vi "GUI_2.vi"() -> ()   [LabVIEW 2023]
uses:
  <vilib>/addons/database/Connection.llb/DB Tools Open Connec (String).vi
  <vilib>/addons/database/Connection.llb/Conn Execute.vi
  <vilib>/addons/database/Recordset.llb/Rec Destroy - Connection.vi
  <vilib>/Instr/_visa.llb/VISA Configure Serial Port (Instr).vi
  <vilib>/addons/database/NI_Database_API.lvlib
panel:
  out "10 V LED":bool
  out "5 V LED":bool
  out "2.5 V LED":bool
  out "1 V LED":bool
  out "10 mV LED":bool
  out "Waveform Graph 2":dbl[](graph)
  in  "stop 2":bool
  out "concatenated string":string
  in  "Unidades":string(combo)
  in  "Canal":enum32{"Item 0", "Item 1"}(radio)
  in  "Guardar":bool
  in  "Autor":string
  out "index":dbl
  out "InicialArr":dbl[](array[numeric])
  out "value":dbl
  out "Canal1":bool
  out "Canal2":bool
  in  "VISA resource name":refnum<visa-resource-name>
  in  "stop":bool
  in  "10 V":bool
  in  "5 V":bool
  in  "2.5 V":bool
  in  "1 V":bool
  in  "10 mV":bool
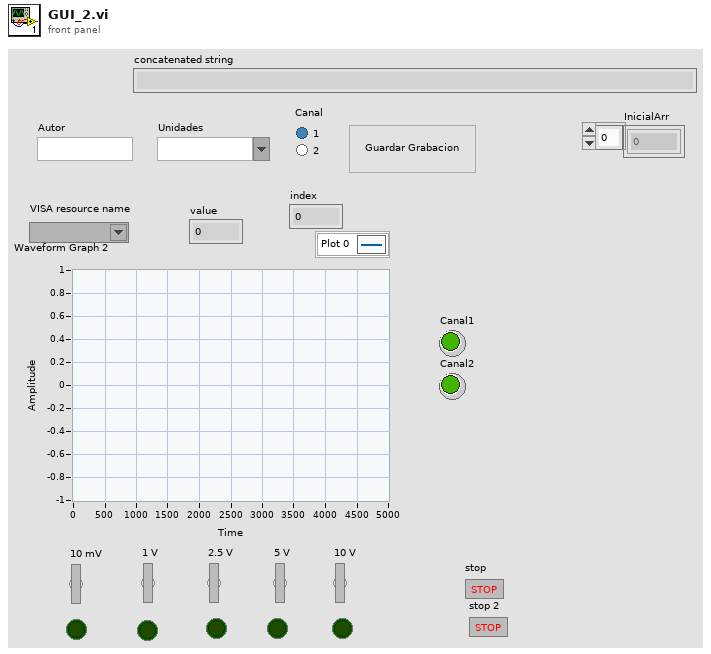
[diagram p1: front panel]
types:
  T1 = typedef "NI_Database_API.lvlib/Conn ObjectReference.ctl" = refnum<k1>
  T2 = typedef "NI_Database_API.lvlib/Rec ObjectReference.ctl" = refnum<k1>
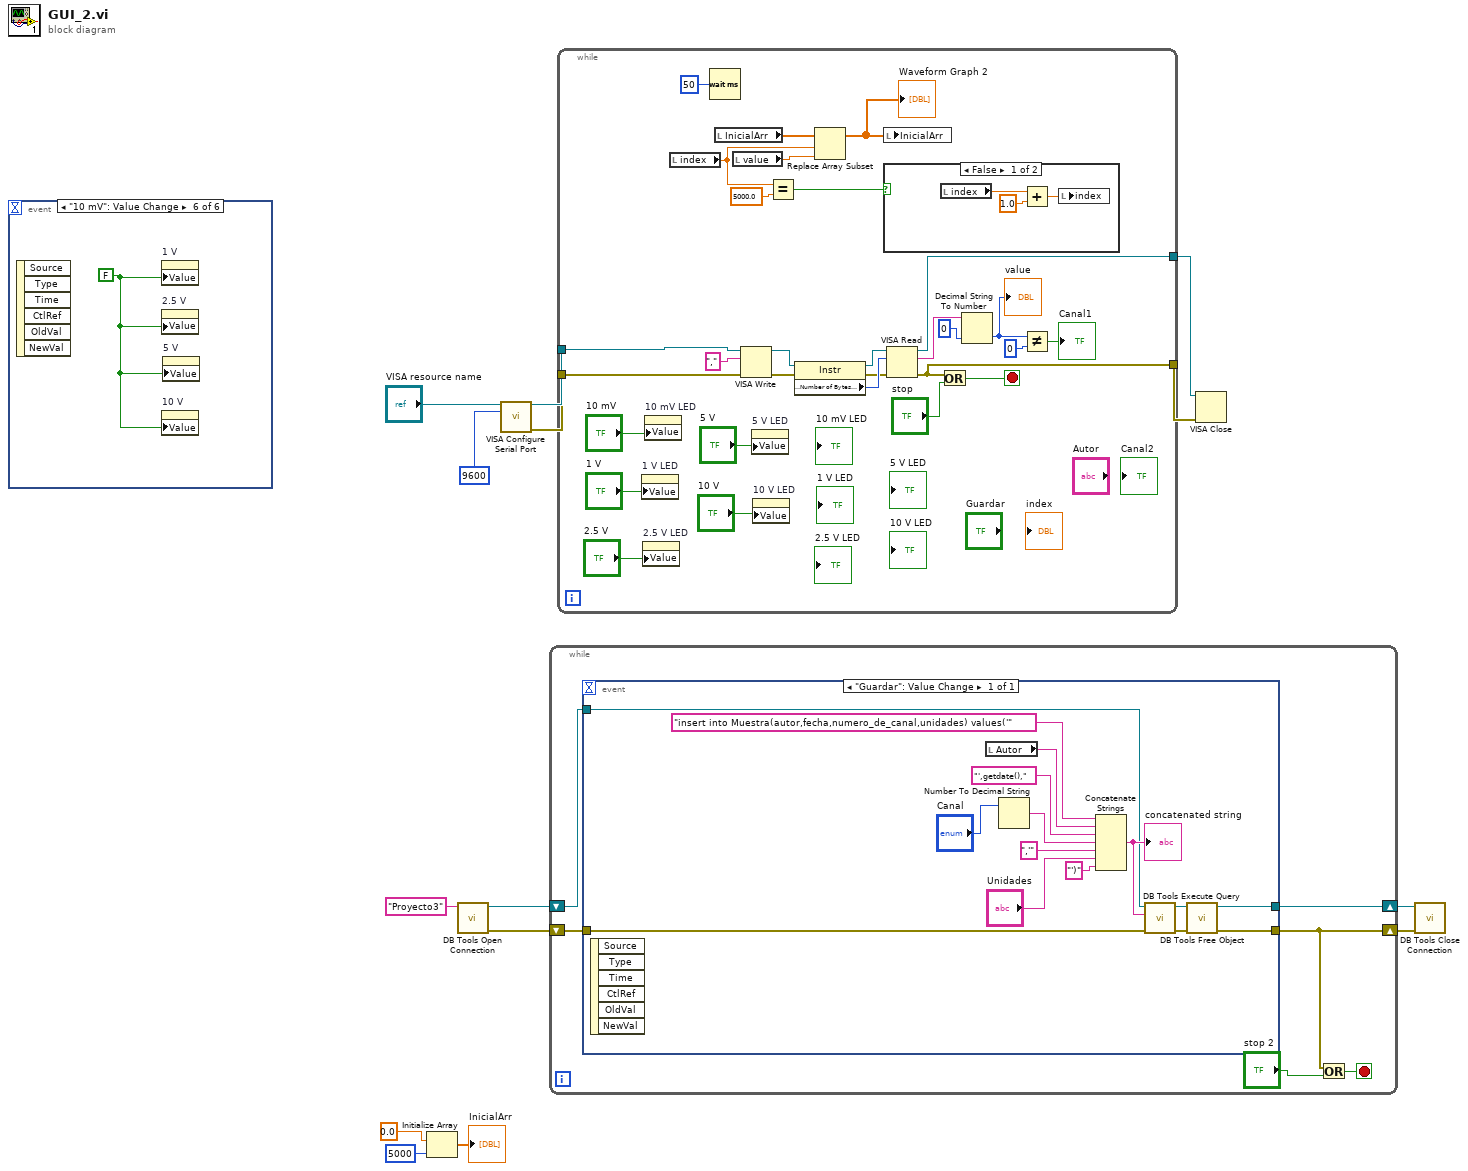
[diagram p0: block diagram]
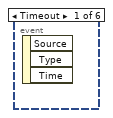
[diagram p2: hidden frame]
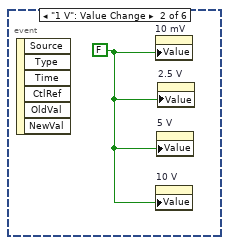
[diagram p3: hidden frame]
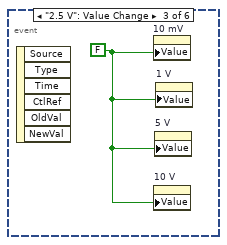
[diagram p4: hidden frame]
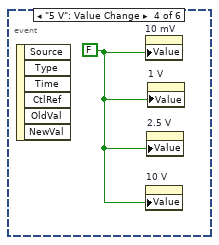
[diagram p5: hidden frame]
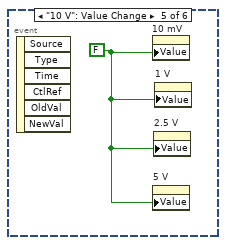
[diagram p6: hidden frame]
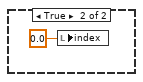
[diagram p7: hidden frame]
diagram:
  n1 = event shown="[5] \"10 mV\": Value Change" {
    selector: _ -> [_ _ _ _ _ _]
    dyn-events: _ -> [_ _ _ _ _ _]
    timeout: _ -> [_ _ _ _ _ _]
    event Timeout {
      n2 = event-data() -> ()  [unwired: 1 in, 3 out]
    }
    event "1 V": Value Change {
      w15 = FALSE
      n3 = event-data() -> ()  [unwired: 1 in, 6 out]
      n4 = property on="10 mV" class="Bool (strict)"("Value"=w15) -> ()  [unwired: 2 in, 2 out]
      n5 = property on="10 V" class="Bool (strict)"("Value"=w15) -> ()  [unwired: 2 in, 2 out]
      n6 = property on="5 V" class="Bool (strict)"("Value"=w15) -> ()  [unwired: 2 in, 2 out]
      n7 = property on="2.5 V" class="Bool (strict)"("Value"=w15) -> ()  [unwired: 2 in, 2 out]
    }
    event "2.5 V": Value Change {
      w16 = FALSE
      n8 = event-data() -> ()  [unwired: 1 in, 6 out]
      n9 = property on="10 mV" class="Bool (strict)"("Value"=w16) -> ()  [unwired: 2 in, 2 out]
      n10 = property on="10 V" class="Bool (strict)"("Value"=w16) -> ()  [unwired: 2 in, 2 out]
      n11 = property on="5 V" class="Bool (strict)"("Value"=w16) -> ()  [unwired: 2 in, 2 out]
      n12 = property on="1 V" class="Bool (strict)"("Value"=w16) -> ()  [unwired: 2 in, 2 out]
    }
    event "5 V": Value Change {
      w17 = FALSE
      n13 = event-data() -> ()  [unwired: 1 in, 6 out]
      n14 = property on="10 mV" class="Bool (strict)"("Value"=w17) -> ()  [unwired: 2 in, 2 out]
      n15 = property on="10 V" class="Bool (strict)"("Value"=w17) -> ()  [unwired: 2 in, 2 out]
      n16 = property on="2.5 V" class="Bool (strict)"("Value"=w17) -> ()  [unwired: 2 in, 2 out]
      n17 = property on="1 V" class="Bool (strict)"("Value"=w17) -> ()  [unwired: 2 in, 2 out]
    }
    event "10 V": Value Change {
      w18 = FALSE
      n18 = event-data() -> ()  [unwired: 1 in, 6 out]
      n19 = property on="10 mV" class="Bool (strict)"("Value"=w18) -> ()  [unwired: 2 in, 2 out]
      n20 = property on="5 V" class="Bool (strict)"("Value"=w18) -> ()  [unwired: 2 in, 2 out]
      n21 = property on="2.5 V" class="Bool (strict)"("Value"=w18) -> ()  [unwired: 2 in, 2 out]
      n22 = property on="1 V" class="Bool (strict)"("Value"=w18) -> ()  [unwired: 2 in, 2 out]
    }
    event "10 mV": Value Change {
      w19 = FALSE
      n23 = event-data() -> ()  [unwired: 1 in, 6 out]
      n24 = property on="1 V" class="Bool (strict)"("Value"=w19) -> ()  [unwired: 2 in, 2 out]
      n25 = property on="2.5 V" class="Bool (strict)"("Value"=w19) -> ()  [unwired: 2 in, 2 out]
      n26 = property on="10 V" class="Bool (strict)"("Value"=w19) -> ()  [unwired: 2 in, 2 out]
      n27 = property on="5 V" class="Bool (strict)"("Value"=w19) -> ()  [unwired: 2 in, 2 out]
    }
  }
  n28 = Initialize Array(0.0 ("element"), 5000 ("dimension size")) -> (→"InicialArr":dbl[])
  n29 = call-poly <vilib>:"DB Tools Open Connection.vi"("connection information"="Proyecto3") -> ("error out"=w4:errorcluster, "connection reference"=w3:T1)  [unwired: 7 in]
  n30 = call-poly "VISA Configure Serial Port"("VISA resource name"="VISA resource name", "baud rate (9600)"=u32 9600) -> ("VISA resource name out"=w14:refnum<visa-resource-name>, "error out"=w11:errorcluster)  [unwired: 12 in]
  n31 = while {
    shift-right: [w21] -> w2
    shift-left: w4 -> [w25]
    shift-right: [w23] -> w1
    shift-left: w3 -> [w24]
    stop <- w22 stop-if-true
    n32 = event shown="[0] \"Guardar\": Value Change" {
      selector: _ -> [_]
      dyn-events: _ -> [_]
      timeout: _ -> [_]
      tunnel: [w29] -> w21
      tunnel: [w28] -> w23
      tunnel: w25 -> [w27]
      tunnel: w24 -> [w26]
      event "Guardar": Value Change {
        n33 = event-data() -> ()  [unwired: 1 in, 6 out]
        n34 = local read "Autor"() -> (w37:string)
        n35 = Number To Decimal String(number="Canal") -> (decimal integer string=w39:string)  [unwired: 1 in]
        n36 = Concatenate Strings("insert into Muestra(autor,fecha,numero_de_canal,unidades) values('", w37, "',getdate(),", w39, ",'" ("string"), "Unidades", "')" ("string")) -> (w40:string)
        "concatenated string" <- w40
        n37 = call-poly <vilib>:"DB Tools Execute Query.vi"("error in (no error)"=w27, "SQL query"=w40, "connection reference"=w26) -> ("error out"=w30:errorcluster, "recordset reference"=w31:T2)  [unwired: 5 in]
        n38 = call-poly <vilib>:"DB Tools Free Object.vi"("error in (no error)"=w30, "recordset reference"=w31) -> ("error out"=w29:errorcluster, "connection reference"=w28:T1)  [unwired: 8 in]
      }
    }
    n39 = Or(x=w21, y="stop 2") -> (x .or. y?=w22:bool)
  }
  n40 = while {
    tunnel: w14 -> [w65]
    tunnel: [w58] -> w13
    tunnel: [w59] -> w12
    tunnel: w11 -> [w63]
    stop <- w47 stop-if-true
    n41 = property on="1 V LED" class="Bool (strict)"("Value"="1 V") -> ()  [unwired: 2 in, 2 out]
    n42 = property on="2.5 V LED" class="Bool (strict)"("Value"="2.5 V") -> ()  [unwired: 2 in, 2 out]
    n43 = property on="10 mV LED" class="Bool (strict)"("Value"="10 mV") -> ()  [unwired: 2 in, 2 out]
    n44 = local read "index"() -> (w53:dbl)
    n45 = Wait (ms)(milliseconds to wait=u32 50) -> ()  [unwired: 1 out]
    n46 = local read "InicialArr"() -> (w52:dbl[])
    n47 = local read "value"() -> (w51:dbl)
    n48 = VISA Write(VISA resource name=w65, write buffer=",", error in (no error)=w63) -> (VISA resource name out=w67:refnum<visa-resource-name>, error out=w62:errorcluster)  [unwired: 1 out]
    n49 = property on="5 V LED" class="Bool (strict)"("Value"="5 V") -> ()  [unwired: 2 in, 2 out]
    n50 = property on="10 V LED" class="Bool (strict)"("Value"="10 V") -> ()  [unwired: 2 in, 2 out]
    n51 = Equal?(x=w53, y=5000.0) -> (x = y?=w54:bool)
    n52 = property class="Instr"(reference=w67, error in=w62) -> (reference out=w66:refnum<visa-resource-name>, error out=w60:errorcluster, "Serial Settings:Number of Bytes at Serial Port"=w61:u32)
    n53 = Replace Array Subset(array=w52, new element=w51, index=w53) -> (w46:dbl[])
    "Waveform Graph 2" <- w46
    n54 = local write "InicialArr"(w46) -> ()
    n55 = case shown="False" w54 {
      frame False {
        n56 = local read "index"() -> (w70:dbl)
        n57 = Add(x=w70, y=1.0 ("index")) -> (x+y=w71:dbl)
        n58 = local write "index"(w71) -> ()
      }
      frame True {
        n59 = local write "index"(0.0 ("index")) -> ()
      }
    }
    n60 = VISA Read(VISA resource name=w66, byte count=w61, error in (no error)=w60) -> (VISA resource name out=w58:refnum<visa-resource-name>, read buffer=w57:string, error out=w59:errorcluster)  [unwired: 1 out]
    n61 = Or(x=w59, y="stop") -> (x .or. y?=w47:bool)
    n62 = Decimal String To Number(string=w57, default (0L)=0 ("default (0 I32)")) -> (number=w50:i32)  [unwired: 1 in, 1 out]
    "value" <- w50
    n63 = Not Equal?(x=w50, y=0) -> (x != y?=→"Canal1":bool)
  }
  n64 = VISA Close(VISA resource name=w13, error in (no error)=w12) -> ()  [unwired: 1 out]
  n65 = call <vilib>:"DB Tools Close Connection.vi"("error in (no error)"=w2, "connection reference"=w1) -> ()  [unwired: 5 in, 1 out]
